vi "Auf Aenderung pruefen.vi"(8 "Gespeicherte Werte":sgl[][](array[numeric]), 11 "Neue Werte":sgl[][](array[numeric])) -> (2 "Änderung?":bool)   [LabVIEW 2020, in "Regler.lvlib" / "Druckregler.lvlib"]
uses:
  Druckregler.lvlib
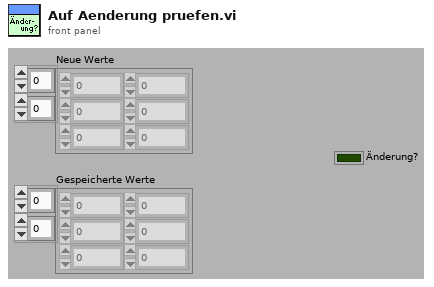
[diagram p1: front panel]
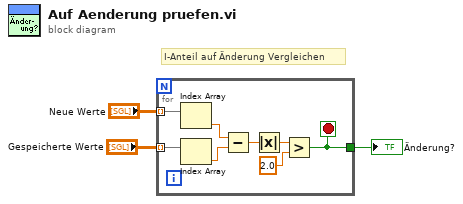
[diagram p0: block diagram]
diagram:
  # "I-Anteil auf Änderung Vergleichen"
  n1 = for {
    tunnel: "Neue Werte" -> [w11] mode=indexing
    tunnel: "Gespeicherte Werte" -> [w10] mode=indexing
    tunnel: [w4] -> w1
    stop <- w4 stop-if-true
    n2 = Index Array(array=w11) -> (element=w9:sgl)  [unwired: 1 in]
    n3 = Index Array(array=w10) -> (element=w8:sgl)  [unwired: 1 in]
    n4 = Subtract(x=w9, y=w8) -> (x-y=w7:sgl)
    n5 = Absolute Value(x=w7) -> (abs(x)=w6:sgl)
    n6 = Greater?(x=w6, y=sgl 2.0) -> (0:w4:bool)
  }
  "Änderung?" <- w1
